vi "14-1.vi"() -> ()   [LabVIEW 2022 SP3, in "AoC22.lvlib"]
uses:
  AoC22.lvlib
  I32Vec2.ctl
  Regolith Cell.ctl
panel:
  in  "Speed":u32(slide)
  out "Resting Sand":i32
  out "Vis":u8[][](graph)
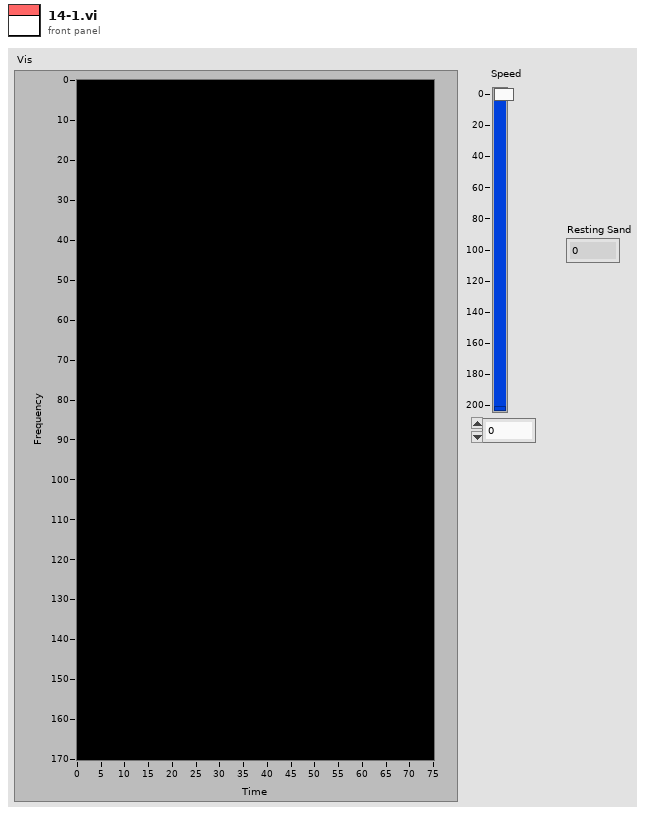
[diagram p1: front panel]
types:
  T1 = typedef "AoC22.lvlib/I32Vec2.ctl" = cluster{"X":i32, "Y":i32}
  T2 = typedef "AoC22.lvlib/Regolith Cell.ctl" = enum16{".", "#", "°", "o", "+"}
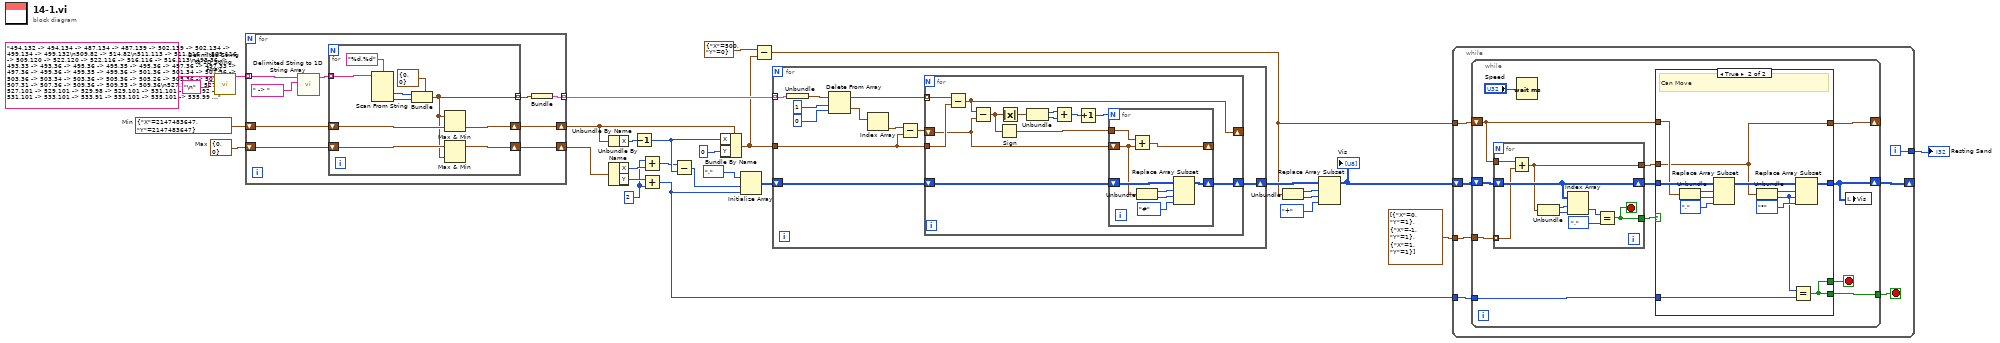
[diagram p0: block diagram]
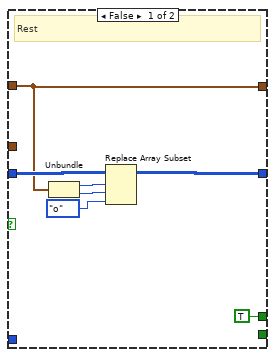
[diagram p2: hidden frame]
diagram:
  w7 = 2 ("y")
  w25 = T1 {"X"=0, "Y"=0}  # Max
  w26 = T1 {"X"=2147483647, "Y"=2147483647}  # Min
  n1 = call <vilib>:"Delimited String to 1D String Array.vi"("delimiter"="\n", "delimited string"="494,132 -> 494,134 -> 487,134 -> 487,139 -> 502,139 -> 502,134 -> 499,134 -> 499,132\n509,82 -> 514,82\n511,113 -> 511,116 -> 509,116 -> 509,120 -> 522,120 -> 522,116 -> 516,116 -> 516,113\n493,36 -> 493,33 -> 493,36 -> 495,36 -> 495,35 -> 495,36 -> 497,36 -> 497,33 -> 497,36 -> 499,36 -> 499,35 -> 499,36 -> 501,36 -> 501,34 -> 501,36 -> 503,36 -> 503,34 -> 503,36 -> 505,36 -> 505,26 -> 505,36 -> 507,36 -> 507,31 -> 507,36 -> 509,36 -> 509,33 -> 509,36\n527,101 -> 527,99 -> 527,101 -> 529,101 -> 529,98 -> 529,101 -> 531,101 -> 531,92 -> 531,101 -> 533,101 -> 533,91 -> 533,101 -> 535,101 -> 535,99 -> 535,101 -> 537,101 -> 537,100 -> 537,101 -> 539,101 -> 539,93 -> 539,101\n493,36 -> 493,33 -> 493,36 -> 495,36 -> 495,35 -> 495,36 -> 497,36 -> 497,33 -> 497,36 -> 499,36 -> 499,35 -> 499,36 -> 501,36 -> 501,34 -> 501,36 -> 503,36 -> 503,34 -> 503,36 -> 505,36 -> 505,26 -> 505,36 -> 507,36 -> 507,31 -> 507,36 -> 509,36 -> 509,33 -> 509,36\n510,65 -> 510,57 -> 510,65 -> 512,65 -> 512,63 -> 512,65 -> 514,65 -> 514,64 -> 514,65\n490,39 -> 490,42 -> 483,42 -> 483,49 -> 503,49 -> 503,42 -> 495,42 -> 495,39\n527,101 -> 527,99 -> 527,101 -> 529,101 -> 529,98 -> 529,101 -> 531,101 -> 531,92 -> 531,101 -> 533,101 -> 533,91 -> 533,101 -> 535,101 -> 535,99 -> 535,101 -> 537,101 -> 537,100 -> 537,101 -> 539,101 -> 539,93 -> 539,101\n526,150 -> 530,150\n493,36 -> 493,33 -> 493,36 -> 495,36 -> 495,35 -> 495,36 -> 497,36 -> 497,33 -> 497,36 -> 499,36 -> 499,35 -> 499,36 -> 501,36 -> 501,34 -> 501,36 -> 503,36 -> 503,34 -> 503,36 -> 505,36 -> 505,26 -> 505,36 -> 507,36 -> 507,31 -> 507,36 -> 509,36 -> 509,33 -> 509,36\n512,127 -> 516,127\n494,132 -> 494,134 -> 487,134 -> 487,139 -> 502,139 -> 502,134 -> 499,134 -> 499,132\n493,36 -> 493,33 -> 493,36 -> 495,36 -> 495,35 -> 495,36 -> 497,36 -> 497,33 -> 497,36 -> 499,36 -> 499,35 -> 499,36 -> 501,36 -> 501,34 -> 501,36 -> 503,36 -> 503,34 -> 503,36 -> 505,36 -> 505,26 -> 505,36 -> 507,36 -> 507,31 -> 507,36 -> 509,36 -> 509,33 -> 509,36\n522,153 -> 522,156 -> 515,156 -> 515,164 -> 533,164 -> 533,156 -> 528,156 -> 528,153\n493,36 -> 493,33 -> 493,36 -> 495,36 -> 495,35 -> 495,36 -> 497,36 -> 497,33 -> 497,36 -> 499,36 -> 499,35 -> 499,36 -> 501,36 -> 501,34 -> 501,36 -> 503,36 -> 503,34 -> 503,36 -> 505,36 -> 505,26 -> 505,36 -> 507,36 -> 507,31 -> 507,36 -> 509,36 -> 509,33 -> 509,36\n517,77 -> 524,77 -> 524,76\n522,153 -> 522,156 -> 515,156 -> 515,164 -> 533,164 -> 533,156 -> 528,156 -> 528,153\n493,36 -> 493,33 -> 493,36 -> 495,36 -> 495,35 -> 495,36 -> 497,36 -> 497,33 -> 497,36 -> 499,36 -> 499,35 -> 499,36 -> 501,36 -> 501,34 -> 501,36 -> 503,36 -> 503,34 -> 503,36 -> 505,36 -> 505,26 -> 505,36 -> 507,36 -> 507,31 -> 507,36 -> 509,36 -> 509,33 -> 509,36\n527,101 -> 527,99 -> 527,101 -> 529,101 -> 529,98 -> 529,101 -> 531,101 -> 531,92 -> 531,101 -> 533,101 -> 533,91 -> 533,101 -> 535,101 -> 535,99 -> 535,101 -> 537,101 -> 537,100 -> 537,101 -> 539,101 -> 539,93 -> 539,101\n529,148 -> 533,148\n521,110 -> 525,110\n493,36 -> 493,33 -> 493,36 -> 495,36 -> 495,35 -> 495,36 -> 497,36 -> 497,33 -> 497,36 -> 499,36 -> 499,35 -> 499,36 -> 501,36 -> 501,34 -> 501,36 -> 503,36 -> 503,34 -> 503,36 -> 505,36 -> 505,26 -> 505,36 -> 507,36 -> 507,31 -> 507,36 -> 509,36 -> 509,33 -> 509,36\n511,113 -> 511,116 -> 509,116 -> 509,120 -> 522,120 -> 522,116 -> 516,116 -> 516,113\n493,36 -> 493,33 -> 493,36 -> 495,36 -> 495,35 -> 495,36 -> 497,36 -> 497,33 -> 497,36 -> 499,36 -> 499,35 -> 499,36 -> 501,36 -> 501,34 -> 501,36 -> 503,36 -> 503,34 -> 503,36 -> 505,36 -> 505,26 -> 505,36 -> 507,36 -> 507,31 -> 507,36 -> 509,36 -> 509,33 -> 509,36\n493,36 -> 493,33 -> 493,36 -> 495,36 -> 495,35 -> 495,36 -> 497,36 -> 497,33 -> 497,36 -> 499,36 -> 499,35 -> 499,36 -> 501,36 -> 501,34 -> 501,36 -> 503,36 -> 503,34 -> 503,36 -> 505,36 -> 505,26 -> 505,36 -> 507,36 -> 507,31 -> 507,36 -> 509,36 -> 509,33 -> 509,36\n506,123 -> 510,123\n490,39 -> 490,42 -> 483,42 -> 483,49 -> 503,49 -> 503,42 -> 495,42 -> 495,39\n494,132 -> 494,134 -> 487,134 -> 487,139 -> 502,139 -> 502,134 -> 499,134 -> 499,132\n522,153 -> 522,156 -> 515,156 -> 515,164 -> 533,164 -> 533,156 -> 528,156 -> 528,153\n522,153 -> 522,156 -> 515,156 -> 515,164 -> 533,164 -> 533,156 -> 528,156 -> 528,153\n527,101 -> 527,99 -> 527,101 -> 529,101 -> 529,98 -> 529,101 -> 531,101 -> 531,92 -> 531,101 -> 533,101 -> 533,91 -> 533,101 -> 535,101 -> 535,99 -> 535,101 -> 537,101 -> 537,100 -> 537,101 -> 539,101 -> 539,93 -> 539,101\n510,65 -> 510,57 -> 510,65 -> 512,65 -> 512,63 -> 512,65 -> 514,65 -> 514,64 -> 514,65\n517,77 -> 524,77 -> 524,76\n520,84 -> 525,84\n506,127 -> 510,127\n522,153 -> 522,156 -> 515,156 -> 515,164 -> 533,164 -> 533,156 -> 528,156 -> 528,153\n494,132 -> 494,134 -> 487,134 -> 487,139 -> 502,139 -> 502,134 -> 499,134 -> 499,132\n494,132 -> 494,134 -> 487,134 -> 487,139 -> 502,139 -> 502,134 -> 499,134 -> 499,132\n497,23 -> 497,14 -> 497,23 -> 499,23 -> 499,16 -> 499,23 -> 501,23 -> 501,17 -> 501,23\n528,88 -> 533,88\n527,101 -> 527,99 -> 527,101 -> 529,101 -> 529,98 -> 529,101 -> 531,101 -> 531,92 -> 531,101 -> 533,101 -> 533,91 -> 533,101 -> 535,101 -> 535,99 -> 535,101 -> 537,101 -> 537,100 -> 537,101 -> 539,101 -> 539,93 -> 539,101\n497,23 -> 497,14 -> 497,23 -> 499,23 -> 499,16 -> 499,23 -> 501,23 -> 501,17 -> 501,23\n493,36 -> 493,33 -> 493,36 -> 495,36 -> 495,35 -> 495,36 -> 497,36 -> 497,33 -> 497,36 -> 499,36 -> 499,35 -> 499,36 -> 501,36 -> 501,34 -> 501,36 -> 503,36 -> 503,34 -> 503,36 -> 505,36 -> 505,26 -> 505,36 -> 507,36 -> 507,31 -> 507,36 -> 509,36 -> 509,33 -> 509,36\n527,101 -> 527,99 -> 527,101 -> 529,101 -> 529,98 -> 529,101 -> 531,101 -> 531,92 -> 531,101 -> 533,101 -> 533,91 -> 533,101 -> 535,101 -> 535,99 -> 535,101 -> 537,101 -> 537,100 -> 537,101 -> 539,101 -> 539,93 -> 539,101\n490,39 -> 490,42 -> 483,42 -> 483,49 -> 503,49 -> 503,42 -> 495,42 -> 495,39\n550,150 -> 554,150\n527,101 -> 527,99 -> 527,101 -> 529,101 -> 529,98 -> 529,101 -> 531,101 -> 531,92 -> 531,101 -> 533,101 -> 533,91 -> 533,101 -> 535,101 -> 535,99 -> 535,101 -> 537,101 -> 537,100 -> 537,101 -> 539,101 -> 539,93 -> 539,101\n493,36 -> 493,33 -> 493,36 -> 495,36 -> 495,35 -> 495,36 -> 497,36 -> 497,33 -> 497,36 -> 499,36 -> 499,35 -> 499,36 -> 501,36 -> 501,34 -> 501,36 -> 503,36 -> 503,34 -> 503,36 -> 505,36 -> 505,26 -> 505,36 -> 507,36 -> 507,31 -> 507,36 -> 509,36 -> 509,33 -> 509,36\n514,88 -> 519,88\n493,36 -> 493,33 -> 493,36 -> 495,36 -> 495,35 -> 495,36 -> 497,36 -> 497,33 -> 497,36 -> 499,36 -> 499,35 -> 499,36 -> 501,36 -> 501,34 -> 501,36 -> 503,36 -> 503,34 -> 503,36 -> 505,36 -> 505,26 -> 505,36 -> 507,36 -> 507,31 -> 507,36 -> 509,36 -> 509,33 -> 509,36\n506,84 -> 511,84\n506,52 -> 512,52 -> 512,51\n516,74 -> 520,74\n524,104 -> 528,104\n506,52 -> 512,52 -> 512,51\n511,113 -> 511,116 -> 509,116 -> 509,120 -> 522,120 -> 522,116 -> 516,116 -> 516,113\n527,106 -> 531,106\n497,23 -> 497,14 -> 497,23 -> 499,23 -> 499,16 -> 499,23 -> 501,23 -> 501,17 -> 501,23\n507,67 -> 507,68 -> 518,68 -> 518,67\n493,36 -> 493,33 -> 493,36 -> 495,36 -> 495,35 -> 495,36 -> 497,36 -> 497,33 -> 497,36 -> 499,36 -> 499,35 -> 499,36 -> 501,36 -> 501,34 -> 501,36 -> 503,36 -> 503,34 -> 503,36 -> 505,36 -> 505,26 -> 505,36 -> 507,36 -> 507,31 -> 507,36 -> 509,36 -> 509,33 -> 509,36\n538,146 -> 542,146\n497,23 -> 497,14 -> 497,23 -> 499,23 -> 499,16 -> 499,23 -> 501,23 -> 501,17 -> 501,23\n515,110 -> 519,110\n527,101 -> 527,99 -> 527,101 -> 529,101 -> 529,98 -> 529,101 -> 531,101 -> 531,92 -> 531,101 -> 533,101 -> 533,91 -> 533,101 -> 535,101 -> 535,99 -> 535,101 -> 537,101 -> 537,100 -> 537,101 -> 539,101 -> 539,93 -> 539,101\n530,108 -> 534,108\n497,23 -> 497,14 -> 497,23 -> 499,23 -> 499,16 -> 499,23 -> 501,23 -> 501,17 -> 501,23\n503,129 -> 507,129\n535,144 -> 539,144\n493,36 -> 493,33 -> 493,36 -> 495,36 -> 495,35 -> 495,36 -> 497,36 -> 497,33 -> 497,36 -> 499,36 -> 499,35 -> 499,36 -> 501,36 -> 501,34 -> 501,36 -> 503,36 -> 503,34 -> 503,36 -> 505,36 -> 505,26 -> 505,36 -> 507,36 -> 507,31 -> 507,36 -> 509,36 -> 509,33 -> 509,36\n493,36 -> 493,33 -> 493,36 -> 495,36 -> 495,35 -> 495,36 -> 497,36 -> 497,33 -> 497,36 -> 499,36 -> 499,35 -> 499,36 -> 501,36 -> 501,34 -> 501,36 -> 503,36 -> 503,34 -> 503,36 -> 505,36 -> 505,26 -> 505,36 -> 507,36 -> 507,31 -> 507,36 -> 509,36 -> 509,33 -> 509,36\n507,67 -> 507,68 -> 518,68 -> 518,67\n500,88 -> 505,88\n507,67 -> 507,68 -> 518,68 -> 518,67\n500,127 -> 504,127\n511,113 -> 511,116 -> 509,116 -> 509,120 -> 522,120 -> 522,116 -> 516,116 -> 516,113\n517,86 -> 522,86\n493,36 -> 493,33 -> 493,36 -> 495,36 -> 495,35 -> 495,36 -> 497,36 -> 497,33 -> 497,36 -> 499,36 -> 499,35 -> 499,36 -> 501,36 -> 501,34 -> 501,36 -> 503,36 -> 503,34 -> 503,36 -> 505,36 -> 505,26 -> 505,36 -> 507,36 -> 507,31 -> 507,36 -> 509,36 -> 509,33 -> 509,36\n497,23 -> 497,14 -> 497,23 -> 499,23 -> 499,16 -> 499,23 -> 501,23 -> 501,17 -> 501,23\n527,110 -> 531,110\n527,101 -> 527,99 -> 527,101 -> 529,101 -> 529,98 -> 529,101 -> 531,101 -> 531,92 -> 531,101 -> 533,101 -> 533,91 -> 533,101 -> 535,101 -> 535,99 -> 535,101 -> 537,101 -> 537,100 -> 537,101 -> 539,101 -> 539,93 -> 539,101\n513,84 -> 518,84\n510,65 -> 510,57 -> 510,65 -> 512,65 -> 512,63 -> 512,65 -> 514,65 -> 514,64 -> 514,65\n533,110 -> 537,110\n503,125 -> 507,125\n535,148 -> 539,148\n507,88 -> 512,88\n493,36 -> 493,33 -> 493,36 -> 495,36 -> 495,35 -> 495,36 -> 497,36 -> 497,33 -> 497,36 -> 499,36 -> 499,35 -> 499,36 -> 501,36 -> 501,34 -> 501,36 -> 503,36 -> 503,34 -> 503,36 -> 505,36 -> 505,26 -> 505,36 -> 507,36 -> 507,31 -> 507,36 -> 509,36 -> 509,33 -> 509,36\n527,101 -> 527,99 -> 527,101 -> 529,101 -> 529,98 -> 529,101 -> 531,101 -> 531,92 -> 531,101 -> 533,101 -> 533,91 -> 533,101 -> 535,101 -> 535,99 -> 535,101 -> 537,101 -> 537,100 -> 537,101 -> 539,101 -> 539,93 -> 539,101\n510,65 -> 510,57 -> 510,65 -> 512,65 -> 512,63 -> 512,65 -> 514,65 -> 514,64 -> 514,65\n524,108 -> 528,108\n490,39 -> 490,42 -> 483,42 -> 483,49 -> 503,49 -> 503,42 -> 495,42 -> 495,39\n527,101 -> 527,99 -> 527,101 -> 529,101 -> 529,98 -> 529,101 -> 531,101 -> 531,92 -> 531,101 -> 533,101 -> 533,91 -> 533,101 -> 535,101 -> 535,99 -> 535,101 -> 537,101 -> 537,100 -> 537,101 -> 539,101 -> 539,93 -> 539,101\n544,150 -> 548,150\n524,86 -> 529,86\n512,80 -> 517,80\n527,101 -> 527,99 -> 527,101 -> 529,101 -> 529,98 -> 529,101 -> 531,101 -> 531,92 -> 531,101 -> 533,101 -> 533,91 -> 533,101 -> 535,101 -> 535,99 -> 535,101 -> 537,101 -> 537,100 -> 537,101 -> 539,101 -> 539,93 -> 539,101\n490,39 -> 490,42 -> 483,42 -> 483,49 -> 503,49 -> 503,42 -> 495,42 -> 495,39\n521,106 -> 525,106\n522,153 -> 522,156 -> 515,156 -> 515,164 -> 533,164 -> 533,156 -> 528,156 -> 528,153\n493,36 -> 493,33 -> 493,36 -> 495,36 -> 495,35 -> 495,36 -> 497,36 -> 497,33 -> 497,36 -> 499,36 -> 499,35 -> 499,36 -> 501,36 -> 501,34 -> 501,36 -> 503,36 -> 503,34 -> 503,36 -> 505,36 -> 505,26 -> 505,36 -> 507,36 -> 507,31 -> 507,36 -> 509,36 -> 509,33 -> 509,36\n527,101 -> 527,99 -> 527,101 -> 529,101 -> 529,98 -> 529,101 -> 531,101 -> 531,92 -> 531,101 -> 533,101 -> 533,91 -> 533,101 -> 535,101 -> 535,99 -> 535,101 -> 537,101 -> 537,100 -> 537,101 -> 539,101 -> 539,93 -> 539,101\n503,86 -> 508,86\n497,23 -> 497,14 -> 497,23 -> 499,23 -> 499,16 -> 499,23 -> 501,23 -> 501,17 -> 501,23\n509,125 -> 513,125\n527,101 -> 527,99 -> 527,101 -> 529,101 -> 529,98 -> 529,101 -> 531,101 -> 531,92 -> 531,101 -> 533,101 -> 533,91 -> 533,101 -> 535,101 -> 535,99 -> 535,101 -> 537,101 -> 537,100 -> 537,101 -> 539,101 -> 539,93 -> 539,101\n532,146 -> 536,146\n516,82 -> 521,82\n510,65 -> 510,57 -> 510,65 -> 512,65 -> 512,63 -> 512,65 -> 514,65 -> 514,64 -> 514,65\n493,36 -> 493,33 -> 493,36 -> 495,36 -> 495,35 -> 495,36 -> 497,36 -> 497,33 -> 497,36 -> 499,36 -> 499,35 -> 499,36 -> 501,36 -> 501,34 -> 501,36 -> 503,36 -> 503,34 -> 503,36 -> 505,36 -> 505,26 -> 505,36 -> 507,36 -> 507,31 -> 507,36 -> 509,36 -> 509,33 -> 509,36\n509,129 -> 513,129\n541,148 -> 545,148\n490,39 -> 490,42 -> 483,42 -> 483,49 -> 503,49 -> 503,42 -> 495,42 -> 495,39\n494,132 -> 494,134 -> 487,134 -> 487,139 -> 502,139 -> 502,134 -> 499,134 -> 499,132\n497,23 -> 497,14 -> 497,23 -> 499,23 -> 499,16 -> 499,23 -> 501,23 -> 501,17 -> 501,23\n493,36 -> 493,33 -> 493,36 -> 495,36 -> 495,35 -> 495,36 -> 497,36 -> 497,33 -> 497,36 -> 499,36 -> 499,35 -> 499,36 -> 501,36 -> 501,34 -> 501,36 -> 503,36 -> 503,34 -> 503,36 -> 505,36 -> 505,26 -> 505,36 -> 507,36 -> 507,31 -> 507,36 -> 509,36 -> 509,33 -> 509,36\n511,113 -> 511,116 -> 509,116 -> 509,120 -> 522,120 -> 522,116 -> 516,116 -> 516,113\n490,39 -> 490,42 -> 483,42 -> 483,49 -> 503,49 -> 503,42 -> 495,42 -> 495,39\n541,144 -> 545,144\n493,36 -> 493,33 -> 493,36 -> 495,36 -> 495,35 -> 495,36 -> 497,36 -> 497,33 -> 497,36 -> 499,36 -> 499,35 -> 499,36 -> 501,36 -> 501,34 -> 501,36 -> 503,36 -> 503,34 -> 503,36 -> 505,36 -> 505,26 -> 505,36 -> 507,36 -> 507,31 -> 507,36 -> 509,36 -> 509,33 -> 509,36\n493,36 -> 493,33 -> 493,36 -> 495,36 -> 495,35 -> 495,36 -> 497,36 -> 497,33 -> 497,36 -> 499,36 -> 499,35 -> 499,36 -> 501,36 -> 501,34 -> 501,36 -> 503,36 -> 503,34 -> 503,36 -> 505,36 -> 505,26 -> 505,36 -> 507,36 -> 507,31 -> 507,36 -> 509,36 -> 509,33 -> 509,36\n511,113 -> 511,116 -> 509,116 -> 509,120 -> 522,120 -> 522,116 -> 516,116 -> 516,113\n538,150 -> 542,150\n510,65 -> 510,57 -> 510,65 -> 512,65 -> 512,63 -> 512,65 -> 514,65 -> 514,64 -> 514,65\n511,113 -> 511,116 -> 509,116 -> 509,120 -> 522,120 -> 522,116 -> 516,116 -> 516,113\n527,101 -> 527,99 -> 527,101 -> 529,101 -> 529,98 -> 529,101 -> 531,101 -> 531,92 -> 531,101 -> 533,101 -> 533,91 -> 533,101 -> 535,101 -> 535,99 -> 535,101 -> 537,101 -> 537,100 -> 537,101 -> 539,101 -> 539,93 -> 539,101\n515,129 -> 519,129\n493,36 -> 493,33 -> 493,36 -> 495,36 -> 495,35 -> 495,36 -> 497,36 -> 497,33 -> 497,36 -> 499,36 -> 499,35 -> 499,36 -> 501,36 -> 501,34 -> 501,36 -> 503,36 -> 503,34 -> 503,36 -> 505,36 -> 505,26 -> 505,36 -> 507,36 -> 507,31 -> 507,36 -> 509,36 -> 509,33 -> 509,36\n510,65 -> 510,57 -> 510,65 -> 512,65 -> 512,63 -> 512,65 -> 514,65 -> 514,64 -> 514,65\n522,153 -> 522,156 -> 515,156 -> 515,164 -> 533,164 -> 533,156 -> 528,156 -> 528,153\n493,36 -> 493,33 -> 493,36 -> 495,36 -> 495,35 -> 495,36 -> 497,36 -> 497,33 -> 497,36 -> 499,36 -> 499,35 -> 499,36 -> 501,36 -> 501,34 -> 501,36 -> 503,36 -> 503,34 -> 503,36 -> 505,36 -> 505,26 -> 505,36 -> 507,36 -> 507,31 -> 507,36 -> 509,36 -> 509,33 -> 509,36\n510,86 -> 515,86\n527,101 -> 527,99 -> 527,101 -> 529,101 -> 529,98 -> 529,101 -> 531,101 -> 531,92 -> 531,101 -> 533,101 -> 533,91 -> 533,101 -> 535,101 -> 535,99 -> 535,101 -> 537,101 -> 537,100 -> 537,101 -> 539,101 -> 539,93 -> 539,101\n494,132 -> 494,134 -> 487,134 -> 487,139 -> 502,139 -> 502,134 -> 499,134 -> 499,132\n521,88 -> 526,88\n527,101 -> 527,99 -> 527,101 -> 529,101 -> 529,98 -> 529,101 -> 531,101 -> 531,92 -> 531,101 -> 533,101 -> 533,91 -> 533,101 -> 535,101 -> 535,99 -> 535,101 -> 537,101 -> 537,100 -> 537,101 -> 539,101 -> 539,93 -> 539,101\n510,65 -> 510,57 -> 510,65 -> 512,65 -> 512,63 -> 512,65 -> 514,65 -> 514,64 -> 514,65\n497,129 -> 501,129\n527,101 -> 527,99 -> 527,101 -> 529,101 -> 529,98 -> 529,101 -> 531,101 -> 531,92 -> 531,101 -> 533,101 -> 533,91 -> 533,101 -> 535,101 -> 535,99 -> 535,101 -> 537,101 -> 537,100 -> 537,101 -> 539,101 -> 539,93 -> 539,101\n532,150 -> 536,150\n493,36 -> 493,33 -> 493,36 -> 495,36 -> 495,35 -> 495,36 -> 497,36 -> 497,33 -> 497,36 -> 499,36 -> 499,35 -> 499,36 -> 501,36 -> 501,34 -> 501,36 -> 503,36 -> 503,34 -> 503,36 -> 505,36 -> 505,26 -> 505,36 -> 507,36 -> 507,31 -> 507,36 -> 509,36 -> 509,33 -> 509,36\n527,101 -> 527,99 -> 527,101 -> 529,101 -> 529,98 -> 529,101 -> 531,101 -> 531,92 -> 531,101 -> 533,101 -> 533,91 -> 533,101 -> 535,101 -> 535,99 -> 535,101 -> 537,101 -> 537,100 -> 537,101 -> 539,101 -> 539,93 -> 539,101\n547,148 -> 551,148\n493,36 -> 493,33 -> 493,36 -> 495,36 -> 495,35 -> 495,36 -> 497,36 -> 497,33 -> 497,36 -> 499,36 -> 499,35 -> 499,36 -> 501,36 -> 501,34 -> 501,36 -> 503,36 -> 503,34 -> 503,36 -> 505,36 -> 505,26 -> 505,36 -> 507,36 -> 507,31 -> 507,36 -> 509,36 -> 509,33 -> 509,36\n518,108 -> 522,108\n544,146 -> 548,146\n527,101 -> 527,99 -> 527,101 -> 529,101 -> 529,98 -> 529,101 -> 531,101 -> 531,92 -> 531,101 -> 533,101 -> 533,91 -> 533,101 -> 535,101 -> 535,99 -> 535,101 -> 537,101 -> 537,100 -> 537,101 -> 539,101 -> 539,93 -> 539,101\n538,142 -> 542,142") -> ("string array"=w27:string[])  [unwired: 9 in]
  n2 = for {
    tunnel: w27 -> [w38] mode=indexing
    tunnel: [w34] -> w20 mode=indexing
    shift-right: [w31] -> w22
    shift-left: w26 -> [w32]
    shift-right: [w30] -> w24
    shift-left: w25 -> [w33]
    n3 = call <vilib>:"Delimited String to 1D String Array.vi"("delimiter"=" -> ", "delimited string"=w38) -> ("string array"=w36:string[])  [unwired: 9 in]
    n4 = for {
      tunnel: w36 -> [w48] mode=indexing
      tunnel: [w40] -> w35 mode=indexing
      shift-right: [w39] -> w30
      shift-left: w33 -> [w41]
      shift-right: [w42] -> w31
      shift-left: w32 -> [w43]
      n5 = Scan From String(format string="%d,%d", input string=w48) -> (output 1=w45:i32, output 2=w44:i32)  [unwired: 4 in, 3 out]
      n6 = Bundle(cluster=T1 {"X"=0, "Y"=0} ("I32Vec2"), "X"=w45, "Y"=w44) -> (w40:T1)
      n7 = Max & Min(x=w40, y=w43) -> (min(x,y)=w42:T1)  [unwired: 1 out]
      n8 = Max & Min(x=w41, y=w40) -> (max(x,y)=w39:T1)  [unwired: 1 out]
    }
    n9 = Bundle(w35) -> (w34:cluster{T1[]})  [unwired: 1 in]
  }
  n10 = Unbundle By Name(w22) -> ("X"=w23:i32)
  n11 = Unbundle By Name(w24) -> ("X"=w9:i32, "Y"=w8:i32)
  n12 = Decrement(x=w23) -> (x-1=w15:i32)
  n13 = Add(x=w7, y=w9) -> (x+y=w6:i32)
  n14 = Add(x=w8, y=w7) -> (x+y=w3:i32)
  n15 = Subtract(x=w6, y=w15) -> (x-y=w18:i32)
  n16 = Bundle By Name(cluster=w22, "X"=w15, "Y"=0) -> (w13:T1)
  n17 = Initialize Array(Regolith_Cell."." ("Regolith Cell"), w18, w3) -> (w17:T2[][])
  n18 = Subtract(x=T1 {"X"=500, "Y"=0} ("I32Vec2"), y=w13) -> (x-y=w1:T1)
  n19 = for {
    tunnel: w13 -> [w51]
    tunnel: w20 -> [w59] mode=indexing
    shift-right: [w56] -> w16
    shift-left: w17 -> [w57]
    n20 = Unbundle(w59) -> (w58:T1[])
    n21 = Delete From Array(array=w58, length=1, index=0) -> (deleted portion=w52:T1[], array with subset deleted=w55:T1[])
    n22 = Index Array(array=w52) -> (element=w49:T1)  [unwired: 1 in]
    n23 = Subtract(x=w49, y=w51) -> (x-y=w50:T1)
    n24 = for {
      tunnel: w55 -> [w72] mode=indexing
      tunnel: w51 -> [w62]
      shift-right: [w70] -> w56
      shift-left: w57 -> [w71]
      shift-right: [w69] -> _
      shift-left: w50 -> [w60]
      n25 = Subtract(x=w72, y=w62) -> (x-y=w69:T1)
      n26 = Subtract(x=w69, y=w60) -> (x-y=w68:T1)
      n27 = Sign(1:w68) -> (0:w61:T1)
      n28 = Absolute Value(x=w68) -> (abs(x)=w67:T1)
      n29 = Unbundle(w67) -> ("X"=w66:i32, "Y"=w65:i32)
      n30 = Add(x=w66, y=w65) -> (x+y=w64:i32)
      n31 = Increment(x=w64) -> (x+1=w63:i32)
      n32 = for {
        N: w63 -> [_]
        shift-right: [w78] -> w70
        shift-left: w71 -> [w80]
        shift-right: [w73] -> _
        shift-left: w60 -> [w75]
        tunnel: w61 -> [w74]
        n33 = Add(x=w74, y=w75) -> (x+y=w73:T1)
        n34 = Unbundle(w75) -> ("X"=w77:i32, "Y"=w76:i32)
        n35 = Replace Array Subset(array=w80, new element=Regolith_Cell."#" ("new element/subarray"), index (row)=w77, index (col)=w76) -> (w78:T2[][])
      }
    }
  }
  n36 = Unbundle(w1) -> ("X"=w12:i32, "Y"=w11:i32)
  n37 = Replace Array Subset(array=w16, new element=Regolith_Cell."+" ("new element/subarray"), index (row)=w12, index (col)=w11) -> (w5:T2[][])
  "Vis" <- w5
  n38 = while {
    shift-right: [w81] -> _
    shift-left: w5 -> [w85]
    tunnel: T1[] [{"X"=0, "Y"=1}, {"X"=-1, "Y"=1}, {"X"=1, "Y"=1}] -> [w84]
    tunnel: w3 -> [w83]
    tunnel: w1 -> [w86]
    tunnel: [w87] -> w2
    i -> [w87]
    stop <- w82 stop-if-true
    n39 = while {
      shift-right: [w89] -> w81
      shift-left: w85 -> [w99]
      tunnel: w84 -> [w98]
      tunnel: w83 -> [w93]
      shift-right: [w90] -> _
      shift-left: w86 -> [w94]
      tunnel: [w92] -> w82
      stop <- w91 stop-if-true
      n40 = for {
        tunnel: w94 -> [w123]
        shift-right: [w126] -> w95
        shift-left: w99 -> [w126]
        tunnel: w98 -> [w122] mode=indexing
        tunnel: [w121] -> w97
        tunnel: [w120] -> w96
        stop <- w121 stop-if-true
        n41 = Add(x=w123, y=w122) -> (x+y=w120:T1)
        n42 = Unbundle(w120) -> ("X"=w128:i32, "Y"=w127:i32)
        n43 = Index Array(array=w126, index (row)=w128, index (col)=w127) -> (element=w125:T2)
        n44 = Equal?(x=w125, y=Regolith_Cell.".") -> (x = y?=w121:bool)
      }
      n45 = Wait (ms)(milliseconds to wait="Speed") -> ()  [unwired: 1 out]
      n46 = case shown="True" w97 {
        tunnel: w96 -> [_ w107]
        tunnel: w95 -> [w103 w119]
        tunnel: w94 -> [w102 w116]
        tunnel: [w100 w111] -> w89
        tunnel: w93 -> [_ w110]
        tunnel: [_ w108] -> w92
        tunnel: [TRUE w108] -> w91
        tunnel: [w102 w107] -> w90
        frame False {
          # "Rest"
          n47 = Unbundle(w102) -> ("X"=w105:i32, "Y"=w104:i32)
          n48 = Replace Array Subset(array=w103, new element=Regolith_Cell."o" ("new element/subarray"), index (row)=w105, index (col)=w104) -> (w100:T2[][])
        }
        frame True {
          # "Can Move"
          n49 = Unbundle(w116) -> ("X"=w118:i32, "Y"=w117:i32)
          n50 = Replace Array Subset(array=w119, new element=Regolith_Cell."." ("new element/subarray"), index (row)=w118, index (col)=w117) -> (w112:T2[][])
          n51 = Unbundle(w107) -> ("X"=w113:i32, "Y"=w109:i32)
          n52 = Equal?(x=w109, y=w110) -> (x = y?=w108:bool)
          n53 = Replace Array Subset(array=w112, new element=Regolith_Cell."°" ("new element/subarray"), index (row)=w113, index (col)=w109) -> (w111:T2[][])
        }
      }
      n54 = local write "Vis"(w89) -> ()
    }
  }
  "Resting Sand" <- w2
